vi "Palette.vi"() -> ()   [LabVIEW 2014, in "SmartPalette.lvlib"]
uses:
  SmartPalette.lvlib
  Controls/QueueDatatype.ctl
  Controls/DataCluster.ctl
  Controls/Palette Data.ctl
  <vilib>/picture/picture.llb/imagedata.ctl
  <vilib>/Utility/miscctls.llb/LVBoundsTypeDef.ctl
  Controls/VI Information.ctl
  <vilib>/Utility/inputDevices.llb/closeMouse.vi
  Usables/Utilities/Error Logger/Error Logger.lvclass
panel:
  in  "Programatic Stop":bool
  out "Header":u32(colorbox) caption="SmartPalette"
  out "2D Picture":picture
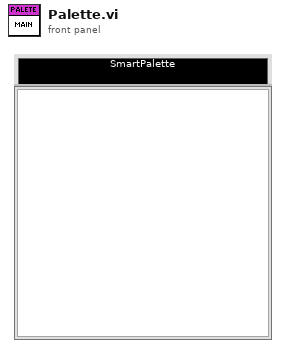
[diagram p1: front panel]
types:
  T1 = typedef "SmartPalette.lvlib/DataCluster.ctl" = cluster{"Monitor VI Name":string, "Read Data":string[], "Display Data":T2[], "DrawBounds":T4}
  T2 = typedef "SmartPalette.lvlib/Palette Data.ctl" = cluster{"PredictedName":string, "PaletteName":string, "ShortName":string, "Pal Icon":T3, "Type":enum16{"SubVI", "Function"}}
  T3 = typedef "imagedata.ctl" = cluster{"image type":i32, "image depth":i32, "image":u8[], "mask":u8[], "colors":u32[], "Rectangle":cluster{"left":i16, "top":i16, "right":i16, "bottom":i16}}
  T4 = typedef "LVBoundsTypeDef.ctl" = cluster{"Width":u32, "Height":u32}
  T5 = typedef "SmartPalette.lvlib/QueueDatatype.ctl" = cluster{"State":string, "Data":variant}
  T6 = enum16{"CreateUsrEvnt", "GenerateUsrEvnt", "GetReference"}
  T7 = enum16{"CreateConnection", "WriteData", "ReadData", "CloseConnection"}
  T8 = typedef "SmartPalette.lvlib/VI Information.ctl" = cluster{"VIAppRef":refnum<vi>, "VIName":string, "Is Block Diagram Active?":bool, "VI Refnum":refnum<vi>}
  T9 = typedef "LVPoint32TypeDef.ctl" = cluster{"Horizontal":i32, "Vertical":i32}
  T10 = typedef "LVPositionTypeDef.ctl" = cluster{"Left":i32, "Top":i32}
  T11 = cluster{"left":i16, "top":i16, "right":i16, "bottom":i16}[]
  T12 = cluster{"left":i16, "top":i16, "right":i16, "bottom":i16}
  T13 = enum32{"Bad", "Idle", "Run top level", "Running"}
  T14 = cluster{"button 1":bool, "button 2":bool, "button 3":bool, "button 4":bool}
  T15 = cluster{"Horizontal":i32, "Vertical":i32, "Scrolling":i32}
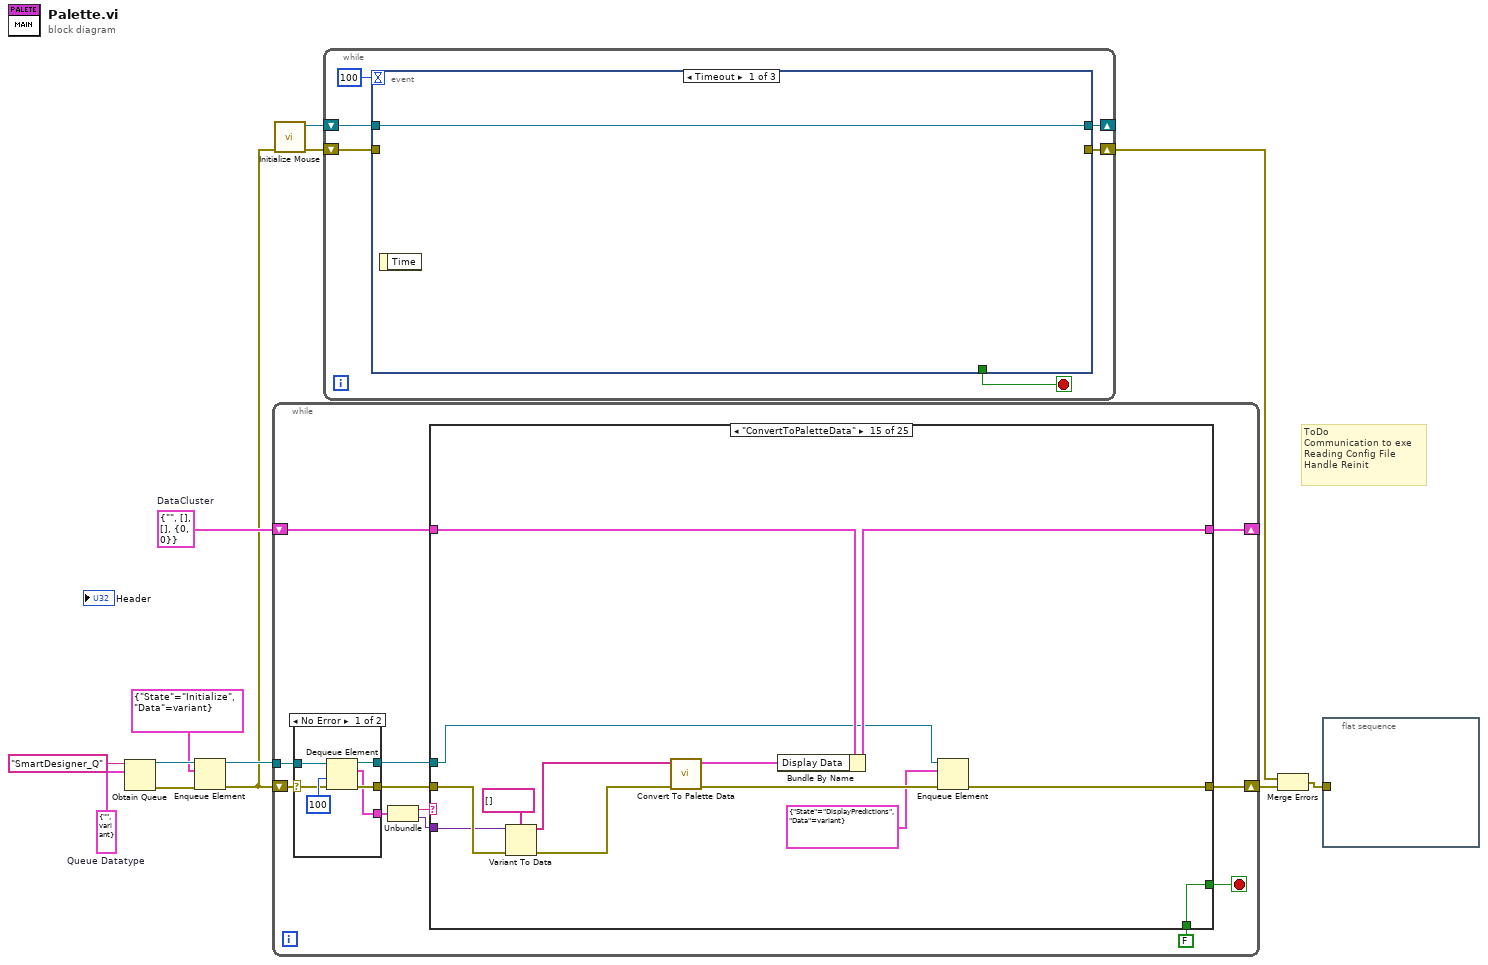
[diagram p0: block diagram]
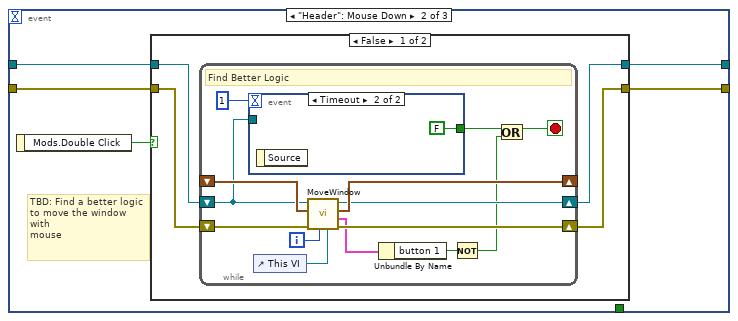
[diagram p2: hidden frame]
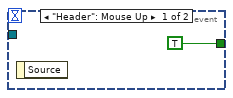
[diagram p3: hidden frame]
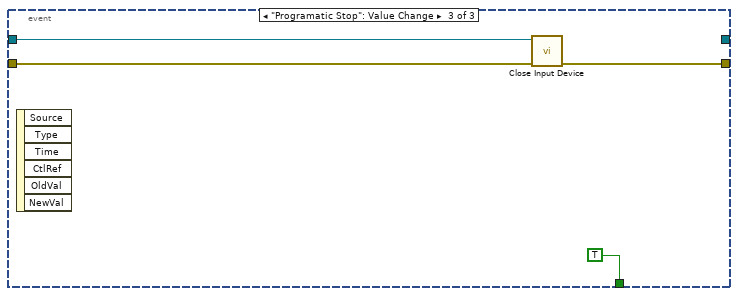
[diagram p5: hidden frame]
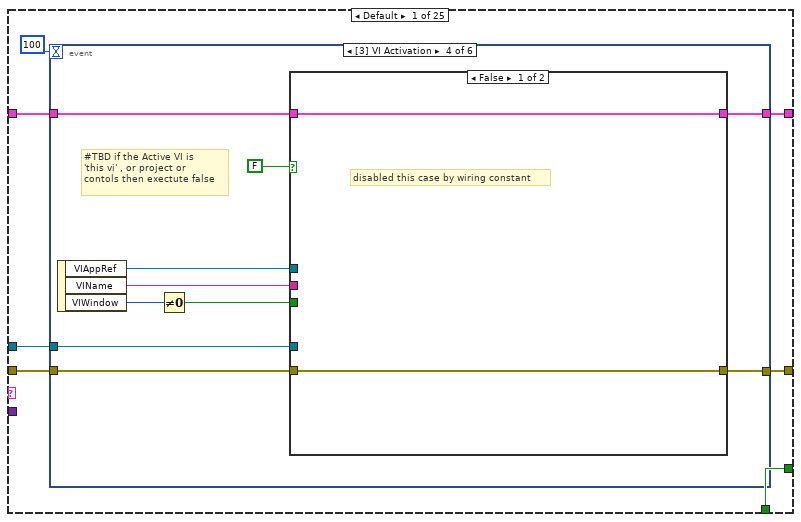
[diagram p6: hidden frame]
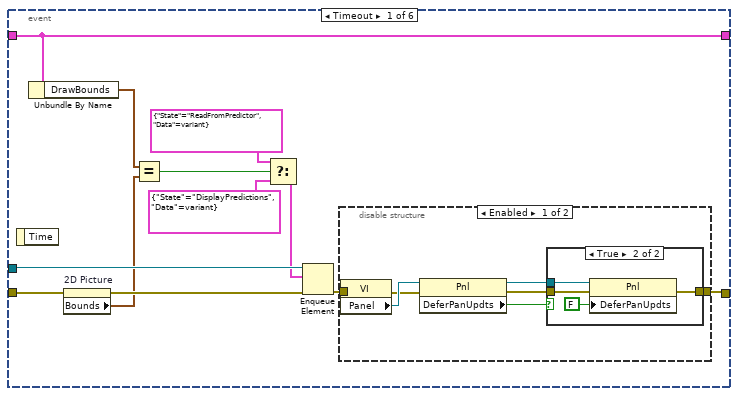
[diagram p7: hidden frame]
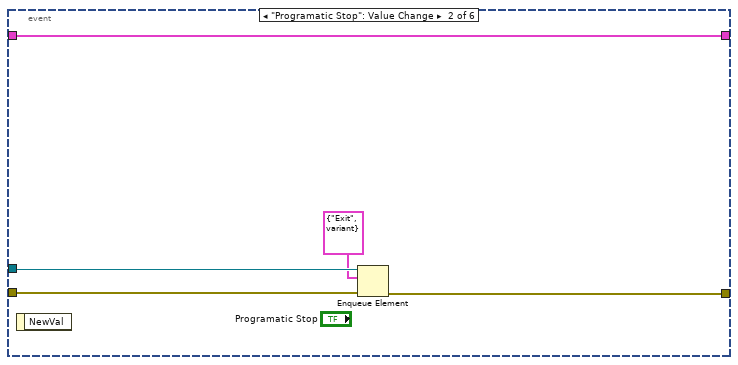
[diagram p10: hidden frame]
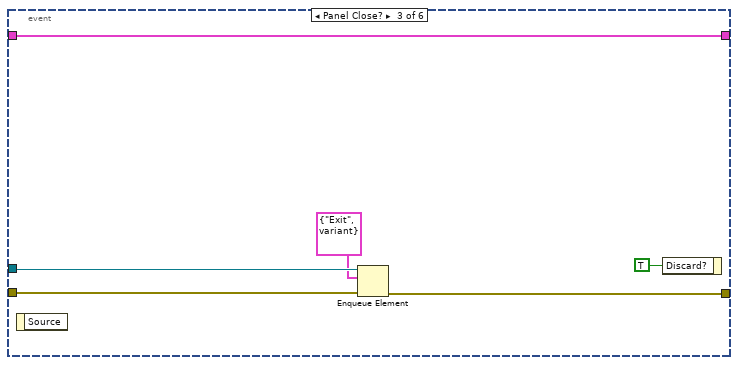
[diagram p11: hidden frame]
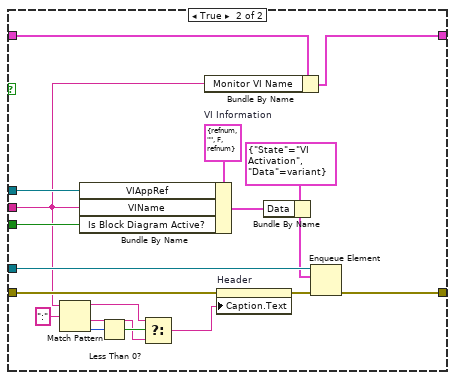
[diagram p12: hidden frame]
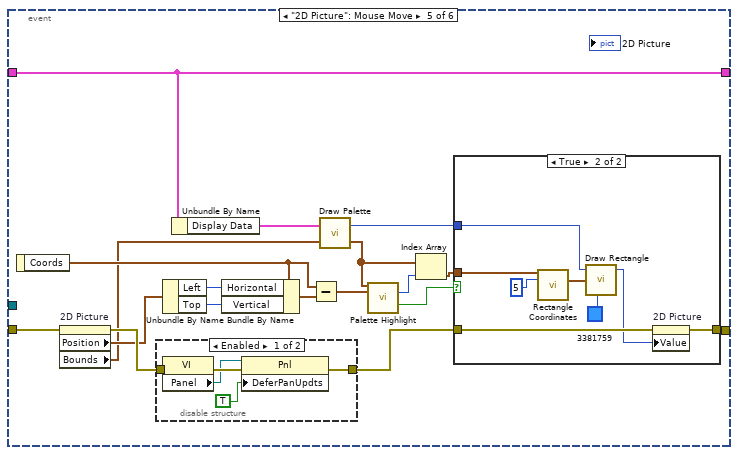
[diagram p13: hidden frame]
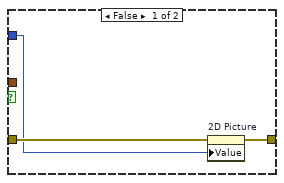
[diagram p15: hidden frame]
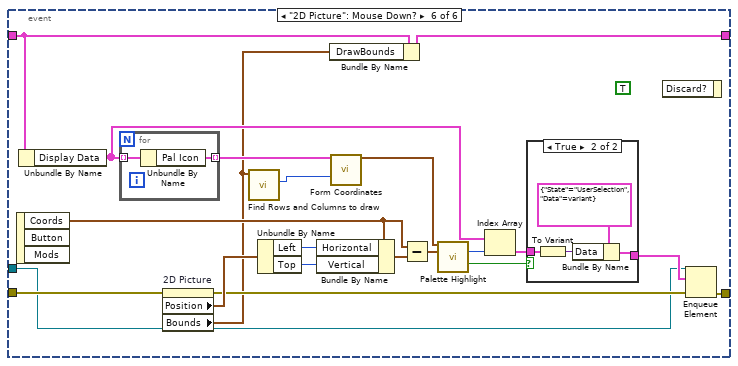
[diagram p16: hidden frame]
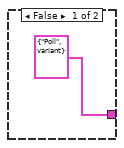
[diagram p17: hidden frame]
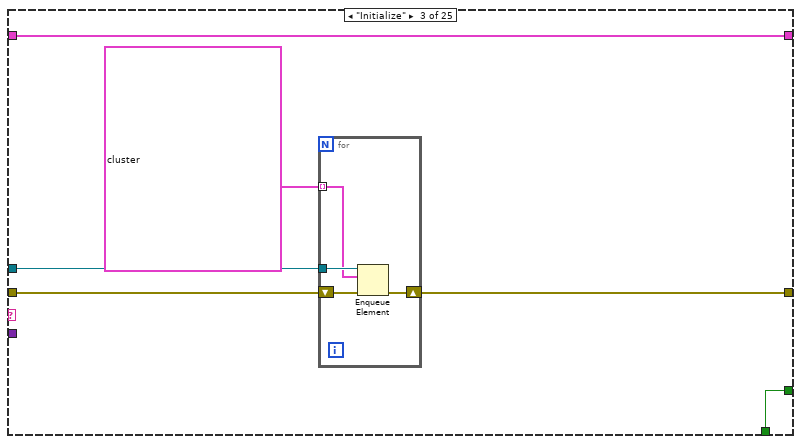
[diagram p19: hidden frame]
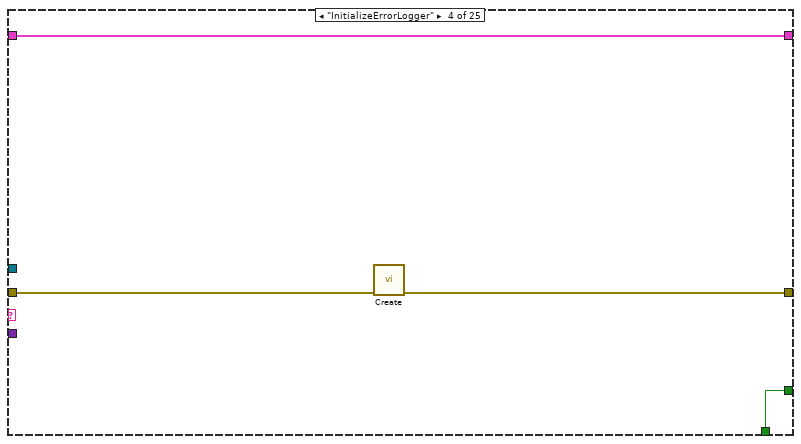
[diagram p20: hidden frame]
diagram:
  w5 = T1 {"Monitor VI Name"="", "Read Data"=[], "Display Data"=[], "DrawBounds"={"Width"=0, "Height"=0}}  # DataCluster
  w13 = T5 {"State"="", "Data"=variant}  # Queue Datatype
  # "ToDo\nCommunication to exe\nReading Config File\nHandle Reinit"
  n1 = Obtain Queue(name (unnamed)="SmartDesigner_Q", element data type=w13) -> (queue out=w11:refnum<queue>, error out=w10:errorcluster)  [unwired: 3 in, 1 out]
  n2 = Enqueue Element(queue=w11, element=T5 {"State"="Initialize", "Data"=variant}, error in (no error)=w10) -> (queue out=w8:refnum<queue>, error out=w1:errorcluster)  [unwired: 1 in, 1 out]
  n3 = while {
    tunnel: w8 -> [w25]
    shift-right: [w17] -> w7
    shift-left: w1 -> [w24]
    shift-right: [w15] -> _
    shift-left: w5 -> [w14]
    stop <- w23 stop-if-true
    n4 = case shown="No Error" w24 {
      selector: w24 -> [w360 w363]
      tunnel: w25 -> [w362 w364]
      tunnel: [w359 w363] -> w16
      tunnel: [w358 w364] -> w18
      tunnel: [w357 T5 {"State"="Error", "Data"=variant} ("Queue Datatype")] -> w21
      frame No Error {
        n5 = Dequeue Element(queue=w362, timeout in ms (-1)=100, error in (no error)=w360) -> (queue out=w358:refnum<queue>, element=w357:T5, error out=w359:errorcluster)  [unwired: 1 out]
      }
      frame Error {
      }
    }
    n6 = Unbundle(w21) -> ("State"=w20:string, "Data"=w19:variant)
    n7 = case shown="\"ConvertToPaletteData\"" w20 {
      tunnel: [w32 w165 w171 w179 w182 w193 w198 w204 w219 w237 w252 w259 w262 w279 w292 w295 w302 w305 w313 w321 w324 w330 w337 w341 TRUE] -> w23
      tunnel: FALSE -> [w32 w165 w171 w179 w182 w193 w198 w204 w219 w237 w252 w259 w262 w279 w292 w295 w302 w305 w313 w321 w324 w330 w337 w341 _]
      tunnel: w19 -> [_ _ _ _ _ _ _ _ _ _ _ w258 _ _ w289 _ _ _ w306 w316 _ _ _ _ _]
      tunnel: w18 -> [w31 _ w170 _ _ _ _ w200 _ _ _ w253 _ w269 w281 _ _ _ w308 _ _ w326 _ _ w352]
      tunnel: [w26 w164 w166 w176 w181 w188 w195 w201 w209 w234 w250 w254 w260 w276 w282 w293 w297 w303 w310 w319 w322 w325 w336 w338 w351] -> w17
      tunnel: w16 -> [w30 w164 w169 w177 w181 w186 w196 w202 w217 w232 w250 w256 w260 w278 w290 w293 w298 w303 w311 w318 w322 w327 w336 w339 w353]
      tunnel: [w27 w163 w167 w178 w180 w184 w197 w203 w218 w236 w251 w255 w261 w264 w285 w294 w301 w304 w312 w320 w323 w329 w335 w340 w350] -> w15
      tunnel: w14 -> [w28 w163 w167 w178 w180 w190 w197 w203 w218 w236 w251 w255 w261 w268 w291 w294 w301 w304 w312 w320 w323 w329 w335 w340 w350]
      frame Default {
        n8 = event shown="[3] VI Activation" {
          selector: _ -> [_ _ _ _ _ _]
          dyn-events: _ -> [_ _ _ _ _ _]
          timeout: 100 -> [_ _ _ _ _ _]
          tunnel: w30 -> [w44 w61 w67 w77 w108 w150]
          tunnel: w31 -> [w43 w62 w68 w76 _ w138]
          tunnel: [w42 w60 w66 w75 w107 w142] -> w26
          tunnel: w28 -> [w37 w58 w63 w71 w105 w148]
          tunnel: [w37 w58 w63 w70 w105 w136] -> w27
          event Timeout {
            n9 = event-data() -> ()  [unwired: 1 in, 1 out]
            n10 = Unbundle By Name(w37) -> ("DrawBounds"=w35:T4)
            n11 = property on="2D Picture" class="Pict"(error in=w44) -> (error out=w36:errorcluster, "Bounds"=w34:T4)  [unwired: 1 in, 1 out]
            n12 = Equal?(x=w35, y=w34) -> (x = y?=w33:bool)
            n13 = Select(t=T5 {"State"="ReadFromPredictor", "Data"=variant} ("element"), s=w33, f=T5 {"State"="DisplayPredictions", "Data"=variant} ("element")) -> (s? t:f=w39:T5)
            n14 = Enqueue Element(queue=w43, element=w39, error in (no error)=w36) -> (error out=w41:errorcluster)  [unwired: 1 in, 2 out]
            n15 = disable-structure shown="Enabled" {
              disable-tunnel: [w46 w57] -> w42
              disable-tunnel: w41 -> [w45 w57]
              frame Enabled {
                n16 = property class="VI"(error in=w45) -> (error out=w50:errorcluster, "Panel"=w51:refnum<vi>)  [unwired: 1 in, 1 out]
                n17 = property class="Pnl"(reference=w51, error in=w50) -> (reference out=w49:refnum<vi>, error out=w48:errorcluster, "DeferPanUpdts"=w47:bool)
                n18 = case shown="True" w47 {
                  tunnel: w49 -> [_ w56]
                  tunnel: w48 -> [w52 w55]
                  tunnel: [w52 w54] -> w46
                  frame False {
                  }
                  frame True {
                    n19 = property class="Pnl"(reference=w56, error in=w55, "DeferPanUpdts"=FALSE) -> (error out=w54:errorcluster)  [unwired: 1 out]
                  }
                }
              }
              frame Disabled {
              }
            }
          }
          event "Programatic Stop": Value Change {
            n20 = event-data() -> ()  [unwired: 1 in, 1 out]
            n21 = Enqueue Element(queue=w62, element=T5 {"State"="Exit", "Data"=variant}, error in (no error)=w61) -> (error out=w60:errorcluster)  [unwired: 1 in, 2 out]
          }
          event Panel Close? {
            n22 = event-data() -> ()  [unwired: 1 in, 1 out]
            n23 = Enqueue Element(queue=w68, element=T5 {"State"="Exit", "Data"=variant}, error in (no error)=w67) -> (error out=w66:errorcluster)  [unwired: 1 in, 2 out]
            n24 = event-data("Discard?"=TRUE) -> ()  [unwired: 1 in, 1 out]
          }
          event VI Activation {
            # "#TBD if the Active VI is\n'this vi' , or project or \ncontols then exectute false"
            n25 = event-data() -> ("VIAppRef"=w73:refnum<vi>, "VIName"=w74:string, "VIWindow"=w78:i32)  [unwired: 1 in]
            n26 = Not Equal To 0?(x=w78) -> (x != 0?=w72:bool)
            n27 = case shown="False" FALSE {
              tunnel: w77 -> [w80 w96]
              tunnel: w76 -> [_ w99]
              tunnel: [w80 w81] -> w75
              tunnel: w74 -> [_ w83]
              tunnel: w73 -> [_ w93]
              tunnel: w72 -> [_ w92]
              tunnel: w71 -> [w79 w84]
              tunnel: [w79 w82] -> w70
              frame False {
                # "disabled this case by wiring constant"
              }
              frame True {
                w94 = T8 {"VIAppRef"=refnum, "VIName"="", "Is Block Diagram Active?"=FALSE, "VI Refnum"=refnum}  # VI Information
                n28 = Match Pattern(string=w83, regular expression=":") -> (before substring=w87:string, after substring=w86:string, offset past match=w89:i32)  [unwired: 1 in, 1 out]
                n29 = Bundle By Name(cluster=w94, "VIAppRef"=w93, "VIName"=w83, "Is Block Diagram Active?"=w92) -> (w91:T8)
                n30 = Less Than 0?(x=w89) -> (x < 0?=w88:bool)
                n31 = Select(t=w87, s=w88, f=w86) -> (s? t:f=w85:string)
                n32 = Bundle By Name(cluster=w84, "Monitor VI Name"=w83) -> (w82:T1)
                n33 = property on="Header" class="ColBox"(error in=w96, "Caption.Text"=w85) -> (error out=w95:errorcluster)  [unwired: 1 in, 1 out]
                n34 = Bundle By Name(cluster=T5 {"State"="VI Activation", "Data"=variant} ("element"), "Data"=w91) -> (w97:T5)
                n35 = Enqueue Element(queue=w99, element=w97, error in (no error)=w95) -> (error out=w81:errorcluster)  [unwired: 1 in, 2 out]
              }
            }
          }
          event "2D Picture": Mouse Move {
            n36 = event-data() -> ("Coords"=w106:T9)  [unwired: 1 in]
            n37 = property on="2D Picture" class="Pict"(error in=w108) -> (error out=w113:errorcluster, "Position"=w109:T10, "Bounds"=w100:T4)  [unwired: 1 in, 1 out]
            n38 = disable-structure shown="Enabled" {
              disable-tunnel: [w121 w123] -> w114
              disable-tunnel: w113 -> [w120 w123]
              frame Enabled {
                n39 = property class="VI"(error in=w120) -> (error out=w119:errorcluster, "Panel"=w118:refnum<vi>)  [unwired: 1 in, 1 out]
                n40 = property class="Pnl"(reference=w118, error in=w119, "DeferPanUpdts"=TRUE) -> (error out=w121:errorcluster)  [unwired: 1 out]
              }
              frame Disabled {
              }
            }
            n41 = Unbundle By Name(w109) -> ("Left"=w110:i32, "Top"=w111:i32)
            n42 = Unbundle By Name(w105) -> ("Display Data"=w104:T2[])
            n43 = Bundle By Name(cluster=w106, "Horizontal"=w110, "Vertical"=w111) -> (w112:T9)
            n44 = Subtract(x=w106, y=w112) -> (x-y=w115:T9)
            n45 = call "Draw Palette.vi"("Bounds  Of Picture"=w100, "Display Data"=w104) -> ("Co-ordinates"=w102:T11, "picture"=w103:picture)
            n46 = call "Palette Highlight.vi"("Co-ordinates"=w102, "Point"=w115) -> ("Index Info"=w116:i32, "Found Palette?"=w101:bool)  [unwired: 12 in]
            n47 = Index Array(array=w102, index=w116) -> (element=w117:T12)
            n48 = case shown="True" w101 {
              tunnel: w114 -> [w126 w133]
              tunnel: w117 -> [_ w129]
              tunnel: [w125 w131] -> w107
              tunnel: w103 -> [w124 w130]
              frame False {
                n49 = property on="2D Picture" class="Pict"(error in=w126, "Value"=w124) -> (error out=w125:errorcluster)  [unwired: 1 in, 1 out]
              }
              frame True {
                n50 = call "Rectangle Coordinates.vi"("Rectangle Coordinates"=w129, "Scaling Factor"=i16 5) -> ("Scaled Rectangle"=w127:T12)  [unwired: 13 in]
                n51 = call <vilib>:"Draw Rectangle.vi"("picture"=w130, "rect"=w127, "color(black)"=u32 3381759) -> ("new picture"=w132:picture)  [unwired: 6 in]
                n52 = property on="2D Picture" class="Pict"(error in=w133, "Value"=w132) -> (error out=w131:errorcluster)  [unwired: 1 in, 1 out]
              }
            }
          }
          event "2D Picture": Mouse Down? {
            (unwired) TRUE ("Discard?")
            n53 = event-data() -> ("Coords"=w151:T9)  [unwired: 1 in, 2 out]
            n54 = Unbundle By Name(w148) -> ("Display Data"=w144:T2[])
            n55 = for {
              tunnel: w144 -> [w162] mode=indexing
              tunnel: [w161] -> w147 mode=indexing
              n56 = Unbundle By Name(w162) -> ("Pal Icon"=w161:T3)
            }
            n57 = property on="2D Picture" class="Pict"(error in=w150) -> (error out=w143:errorcluster, "Position"=w152:T10, "Bounds"=w135:T4)  [unwired: 1 in, 1 out]
            n58 = call "Find Rows and Columns to draw.vi"("Bounds  Of Picture"=w135) -> ("Col"=w137:u32)  [unwired: 8 in, 2 out]
            n59 = Unbundle By Name(w152) -> ("Left"=w155:i32, "Top"=w154:i32)
            n60 = Bundle By Name(cluster=w151, "Horizontal"=w155, "Vertical"=w154) -> (w153:T9)
            n61 = Bundle By Name(cluster=w148, "DrawBounds"=w135) -> (w136:T1)
            n62 = call "Form Coordinates.vi"("Palette Item Icon"=w147, "No.of Elements in Row"=w137) -> ("Co-ordinates"=w146:T11)  [unwired: 13 in]
            n63 = Subtract(x=w151, y=w153) -> (x-y=w149:T9)
            n64 = call "Palette Highlight.vi"("Co-ordinates"=w146, "Point"=w149) -> ("Index Info"=w145:i32, "Found Palette?"=w141:bool)  [unwired: 12 in]
            n65 = Index Array(array=w144, index=w145) -> (element=w140:T2)
            n66 = case shown="True" w141 {
              tunnel: w140 -> [_ w159]
              tunnel: [T5 {"State"="Poll", "Data"=variant} ("element") w157] -> w139
              frame False {
              }
              frame True {
                n67 = To Variant(anything=w159) -> (Variant=w158:variant)
                n68 = Bundle By Name(cluster=T5 {"State"="UserSelection", "Data"=variant} ("element"), "Data"=w158) -> (w157:T5)
              }
            }
            n69 = event-data() -> ()  [unwired: 2 in, 1 out]
            n70 = Enqueue Element(queue=w138, element=w139, error in (no error)=w143) -> (error out=w142:errorcluster)  [unwired: 1 in, 2 out]
          }
        }
      }
      frame "---------------InitializeSequence---------------" {
      }
      frame "Initialize" {
        n71 = for {
          shift-right: [w174] -> w166
          shift-left: w169 -> [w175]
          tunnel: w170 -> [w173]
          tunnel: T5[] [{"State"="InitializeErrorLogger", "Data"=variant}, {"State"="InitializeData", "Data"=variant}, {"State"="InitializeUI", "Data"=variant}, {"State"="InitializeUserEvents", "Data"=variant}, {"State"="InitializeComplete", "Data"=variant}] -> [w172] mode=indexing
          n72 = Enqueue Element(queue=w173, element=w172, error in (no error)=w175) -> (error out=w174:errorcluster)  [unwired: 1 in, 2 out]
        }
      }
      frame "InitializeErrorLogger" {
        n73 = call "Create.vi"("error in"=w177) -> ("error out"=w176:errorcluster)  [unwired: 14 in]
      }
      frame "InitializeData" {
        # "#TBD \n1. Initialize the Data for application\n\n2. get the data from the SmartPalette.ini file and update the cluster\n\n3. one of the parameter can be how many last VI's data to store (in previous version \nuid is stored, i think we can store the last prediction list of previous VI's)\n\n4. ....."
        n74 = call "Read Settings.vi"() -> ()  [unwired: 12 in]
      }
      frame "InitializeUI" {
        # "#TBD\n\n1. Initialize the UI components"
        n75 = property on="2D Picture" class="Pict"(error in=w186) -> (error out=w185:errorcluster, "Bounds"=w183:T4)  [unwired: 1 in, 1 out]
        n76 = Bundle By Name(cluster=w190, "DrawBounds"=w183) -> (w184:T1)
        n77 = property on="Header" class="ColBox"(error in=w185, "Caption.Text"="SmartPalette", "Caption.TextColor"=u32 16777215 ("Header Normal")) -> (error out=w192:errorcluster)  [unwired: 1 in, 1 out]
        n78 = property on="2D Picture" class="Pict"(error in=w192, "Value"=picture data[5B] ("2D Picture")) -> (error out=w188:errorcluster)  [unwired: 1 in, 1 out]
      }
      frame "InitializeUserEvents" {
        n79 = call "Palette UserEvents.vi"("Enum"=T6."CreateUsrEvnt", "error in (no error)"=w196) -> ("error out"=w195:errorcluster)  [unwired: 8 in, 1 out]
      }
      frame "InitializeComplete" {
        n80 = for {
          tunnel: T5[] [{"State"="StartMonitoringVI", "Data"=variant}, {"State"="StartPredictor", "Data"=variant}] -> [w208] mode=indexing
          tunnel: w200 -> [w205]
          shift-right: [w206] -> w201
          shift-left: w202 -> [w207]
          n81 = Enqueue Element(queue=w205, element=w208, error in (no error)=w207) -> (error out=w206:errorcluster)  [unwired: 1 in, 2 out]
        }
      }
      frame "StartMonitoringVI" {
        n82 = call "Get All Paths.vi"("error in"=w217) -> ("Monitor VI path"=w214:path, "error out"=w216:errorcluster)  [unwired: 9 in, 4 out]
        n83 = Open VI Reference(vi path=w214, error in (no error)=w216) -> (vi reference=w213:refnum<vi>, error out=w215:errorcluster)  [unwired: 4 in]
        n84 = property class="VI"(reference=w213, error in=w215) -> (reference out=w210:refnum<vi>, error out=w212:errorcluster, "Exec.State"=w211:T13)
        n85 = case shown="\"Run top level\", \"Running\"" w211 {
          tunnel: w212 -> [w222 w226 w230]
          tunnel: [w222 w225 w229] -> w209
          tunnel: w210 -> [_ w224 _]
          frame "Bad", Default {
            # "ToDo: Remove popup"
            n86 = One Button Dialog(message="Monitoring Vi is in bad state", button name ("OK")="Contiue") -> ()  [unwired: 1 out]
          }
          frame "Idle" {
            n87 = invoke class="VI" method="Run VI"(reference=w224, error in=w226, "Wait until done"=FALSE ("Wait Until Done")) -> (error out=w225:errorcluster)  [unwired: 2 in, 4 out]
          }
          frame "Run top level", "Running" {
            n88 = call "Palette UserEvents.vi"("Enum"=T6."GenerateUsrEvnt", "error in (no error)"=w230, "MainVICommand"="Restart") -> ("error out"=w229:errorcluster)  [unwired: 7 in, 1 out]
          }
        }
      }
      frame "StartPredictor" {
        n89 = disable-structure shown="Enabled" {
          disable-tunnel: w232 -> [w243 w249]
          disable-tunnel: [w244 w249] -> w233
          frame Enabled {
            n90 = flat-sequence {
              tunnel: w243 -> [w247]
              tunnel: [w247] -> w242
              frame #0 {
                n91 = Wait (ms)(milliseconds to wait=u32 1000) -> ()  [unwired: 1 out]
              }
            }
            n92 = call "Get All Paths.vi"("error in"=w242) -> ("Predictor path"=w240:path, "error out"=w245:errorcluster)  [unwired: 9 in, 4 out]
            n93 = Path To String(path=w240) -> (string=w246:string)
            n94 = Strip Path(path=w240) -> (stripped path=w239:path)  [unwired: 1 out]
            n95 = call <vilib>:"System Exec.vi"("run minimized? (F)"=TRUE, "wait until completion? (T)"=FALSE, "error in (no error)"=w245, "working directory"=w239, "command line"=w246) -> ("error out"=w244:errorcluster)  [unwired: 3 in, 3 out]
          }
          frame Disabled {
          }
        }
        n96 = call "TCPCommunication.vi"("error in (no error)"=w232, "Selector"=T7."CreateConnection") -> ("error out"=w231:errorcluster)  [unwired: 12 in, 1 out]
        n97 = Merge Errors(w233, w231) -> (w234:errorcluster)
      }
      frame "----------------Handle Events--------------" {
      }
      frame "VI Activation" {
        # "#TBD\n\n1. See if the Active VI is one of the previously stored VI. if it is read the data and display\n2. or extract the functions by some way (ideas?) and display the prediction for it"
        n98 = Variant To Data(error in=w256, type=T8 {"VIAppRef"=refnum, "VIName"="", "Is Block Diagram Active?"=FALSE, "VI Refnum"=refnum} ("VI Information"), Variant=w258) -> (error out=w254:errorcluster)  [unwired: 1 out]
        n99 = flat-sequence {
          tunnel: w253 -> [_]
          frame #0 {
            # "Enqueue with conditions if needed\n1. ExtractDataforPrediction\n2. Query&GetPredictedList\n3. GetPaletteIcons\n4. DisplayPredictions"
          }
        }
      }
      frame "----------------Operations--------------" {
      }
      frame "ReadFromPredictor" {
        n100 = Unbundle By Name(w268) -> ("Read Data"=w267:string[])
        n101 = call "Read Data From Predictor.vi"("error in (no error)"=w278) -> ("Nodes To Display"=w263:string[], "error out"=w277:errorcluster)  [unwired: 13 in]
        n102 = Empty Array?(array=w263) -> (empty?=w275:bool)
        n103 = Equal?(x=w263, y=w267) -> (x = y?=w265:bool)
        n104 = To Variant(anything=w263) -> (Variant=w270:variant)
        n105 = Bundle By Name(cluster=w268, "Read Data"=w263) -> (w264:T1)
        n106 = Or(x=w265, y=w275) -> (x .or. y?=w266:bool)
        n107 = Bundle By Name(cluster=T5 {"State"="ConvertToPaletteData", "Data"=variant} ("element"), "Data"=w270) -> (w271:T5)
        n108 = Select(t=T5 {"State"="Poll", "Data"=variant} ("element"), s=w266, f=w271) -> (s? t:f=w273:T5)
        n109 = Enqueue Element(queue=w269, element=w273, error in (no error)=w277) -> (error out=w276:errorcluster)  [unwired: 1 in, 2 out]
      }
      frame "ConvertToPaletteData" {
        n110 = Variant To Data(error in=w290, type=string[] [] ("Nodes To Display"), Variant=w289) -> (data=w286:string[], error out=w287:errorcluster)
        n111 = call "Convert To Palette Data.vi"("error in (no error)"=w287, "Predicted Data[]"=w286) -> ("error out"=w283:errorcluster, "Array"=w284:T2[])  [unwired: 8 in]
        n112 = Bundle By Name(cluster=w291, "Display Data"=w284) -> (w285:T1)
        n113 = Enqueue Element(queue=w281, element=T5 {"State"="DisplayPredictions", "Data"=variant}, error in (no error)=w283) -> (error out=w282:errorcluster)  [unwired: 1 in, 2 out]
      }
      frame "---------------------Display---------------------" {
      }
      frame "DisplayPredictions" {
        n114 = Unbundle By Name(w301) -> ("Display Data"=w300:T2[])
        n115 = property on="2D Picture" class="Pict"(error in=w298) -> (error out=w297:errorcluster, "Bounds"=w296:T4)  [unwired: 1 in, 1 out]
        n116 = call "Draw Palette.vi"("Bounds  Of Picture"=w296, "Display Data"=w300) -> ("picture"=w299:picture)  [unwired: 1 out]
        n117 = local write "2D Picture"(w299) -> ()
      }
      frame "-------/*Selection Operartions*/--------" {
      }
      frame "UserSelection" {
        # "ToDo\nAdd cases depends on condition(Keyboard)\n1. Place Node next to new node\n2. place and wire \nand etc"
        n118 = Bundle By Name(cluster=T5 {"State"="BringtoCursor", "Data"=variant} ("element"), "Data"=w306) -> (w307:T5)
        n119 = Enqueue Element(queue=w308, element=w307, error in (no error)=w311) -> (error out=w310:errorcluster)  [unwired: 1 in, 2 out]
      }
      frame "BringtoCursor" {
        n120 = Variant To Data(error in=w318, type=T2 {"PredictedName"="", "PaletteName"="", "ShortName"="", "Pal Icon"={"image type"=0, "image depth"=0, "image"=[], "mask"=[], "colors"=[], "Rectangle"={"left"=0, "top"=0, "right"=0, "bottom"=0}}, "Type"=enum."Function"} ("Palette Data"), Variant=w316) -> (data=w314:T2, error out=w317:errorcluster)
        n121 = call "Bring To Cursor.vi"("error in (no error)"=w317, "Palette Data"=w314) -> ("error out"=w319:errorcluster)  [unwired: 9 in]
      }
      frame "--------------ReInitialize Sequence-------------" {
      }
      frame "HandleReInitialize" {
        # "#TBD\n1. If there is any change in settings use this to update the application\n\nits a place holder for now"
        n122 = for {
          shift-right: [w333] -> w325
          shift-left: w327 -> [w334]
          tunnel: w326 -> [w332]
          tunnel: T5[] [] -> [w331] mode=indexing
          n123 = Enqueue Element(queue=w332, element=w331, error in (no error)=w334) -> (error out=w333:errorcluster)  [unwired: 1 in, 2 out]
        }
      }
      frame "---------------------misc-----------------------" {
      }
      frame "Error" {
        n124 = call "LogError.vi"("error in"=w339) -> ("error out"=w338:errorcluster)  [unwired: 10 in]
      }
      frame "Exit" {
        n125 = Release Queue(queue=w352, error in (no error)=w353) -> (error out=w346:errorcluster)  [unwired: 1 in, 2 out]
        n126 = call "Palette UserEvents.vi"("Enum"=T6."GenerateUsrEvnt", "error in (no error)"=w346, "MainVICommand"="Exit") -> ("error out"=w343:errorcluster)  [unwired: 7 in, 1 out]
        n127 = flat-sequence {
          tunnel: w343 -> [w355]
          tunnel: [w355] -> w342
          frame #0 {
            n128 = Wait (ms)(milliseconds to wait=u32 200) -> ()  [unwired: 1 out]
          }
        }
        n129 = call "TCPCommunication.vi"("error in (no error)"=w342, "Selector"=T7."CloseConnection") -> ("error out"=w344:errorcluster)  [unwired: 12 in, 1 out]
        n130 = Merge Errors(w344) -> (w349:errorcluster)
        n131 = call "Clear.vi"("error in (no error)"=w349) -> ("error out"=w351:errorcluster)  [unwired: 10 in]
      }
    }
  }
  n132 = call <vilib>:"Initialize Mouse.vi"("error in (no error)"=w1) -> ("error out"=w3:errorcluster, "device ID"=w4:refnum<k1>)  [unwired: 9 out]
  n133 = while {
    shift-right: [w369] -> _
    shift-left: w4 -> [w370]
    shift-right: [w367] -> w2
    shift-left: w3 -> [w368]
    stop <- w366 stop-if-true
    n134 = event shown="[0] Timeout" {
      selector: _ -> [_ _ _]
      dyn-events: _ -> [_ _ _]
      timeout: 100 -> [_ _ _]
      tunnel: w370 -> [w372 w376 w402]
      tunnel: [w372 w375 _] -> w369
      tunnel: w368 -> [_ w374 w400]
      tunnel: [_ w373 w401] -> w367
      tunnel: [_ _ TRUE] -> w366
      event Timeout {
        n135 = event-data() -> ()  [unwired: 1 in, 1 out]
      }
      event "Header": Mouse Down {
        # "TBD: Find a better logic\nto move the window with\nmouse"
        n136 = event-data() -> ("Mods.Double Click"=w377:bool)  [unwired: 1 in]
        n137 = case shown="False" w377 {
          tunnel: w376 -> [w381 w399]
          tunnel: [w380 w399] -> w375
          tunnel: w374 -> [w379 w398]
          tunnel: [w378 w398] -> w373
          frame False {
            n138 = while {
              shift-right: [w391] -> w380
              shift-left: w381 -> [w386]
              shift-right: [w394] -> w378
              shift-left: w379 -> [w393]
              shift-right: [w392] -> _
              shift-left: _ -> [w387]
              i -> [w389]
              stop <- w383 stop-if-true
              # "Find Better Logic"
              n139 = event shown="[1] Timeout" {
                selector: _ -> [_ _]
                dyn-events: _ -> [_ _]
                timeout: 1 -> [_ _]
                tunnel: [TRUE FALSE] -> w395
                tunnel: w386 -> [_ _]
                event "Header": Mouse Up {
                  n140 = event-data() -> ()  [unwired: 2 out]
                }
                event Timeout {
                  n141 = event-data() -> ()  [unwired: 2 out]
                }
              }
              n142 = control-ref of="This VI"() -> (w388:refnum<vi>)
              n143 = call "MoveWindow.vi"("Window Reference"=w388, "Iteration"=w389, "error in (no error)"=w393, "axis info in"=w387, "Refnum in"=w386) -> ("error out"=w394:errorcluster, "button info"=w385:T14, "axis info"=w392:T15, "Refnum out"=w391:refnum<k1>)  [unwired: 3 in]
              n144 = Unbundle By Name(w385) -> ("button 1"=w384:bool)
              n145 = Not(x=w384) -> (.not. x?=w382:bool)
              n146 = Or(x=w395, y=w382) -> (x .or. y?=w383:bool)
            }
          }
          frame True {
          }
        }
      }
      event "Programatic Stop": Value Change {
        n147 = event-data() -> ()  [unwired: 1 in, 6 out]
        n148 = call-poly <vilib>:"Close Input Device.vi"("error in (no error)"=w400, "device ID"=w402) -> ("error out"=w401:errorcluster)  [unwired: 8 out]
      }
    }
  }
  n149 = Merge Errors(w2, w7) -> (w6:errorcluster)
  n150 = flat-sequence {
    tunnel: w6 -> [_]
    frame #0 {
    }
  }
